vi "lookupImage.vi"(8 "error in (no error)":errorcluster, 11 "ImageStreamViewer in":refnum<class "ImageStreamViewer.lvclass">) -> (0 "error out":errorcluster, 3 "ImageStreamViewer out":refnum<class "ImageStreamViewer.lvclass">)   [LabVIEW 2009, in "Views.lvlib" / "Camera.lvlib" / "ImageStreamViewer.lvclass"]
uses:
  ImageStreamViewer.lvclass
  ImageStreamViewer.lvclass/ImageStreamViewer.ctl
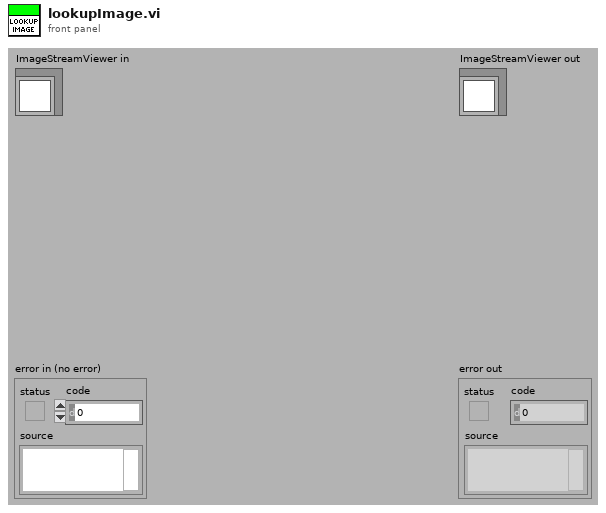
[diagram p1: front panel]
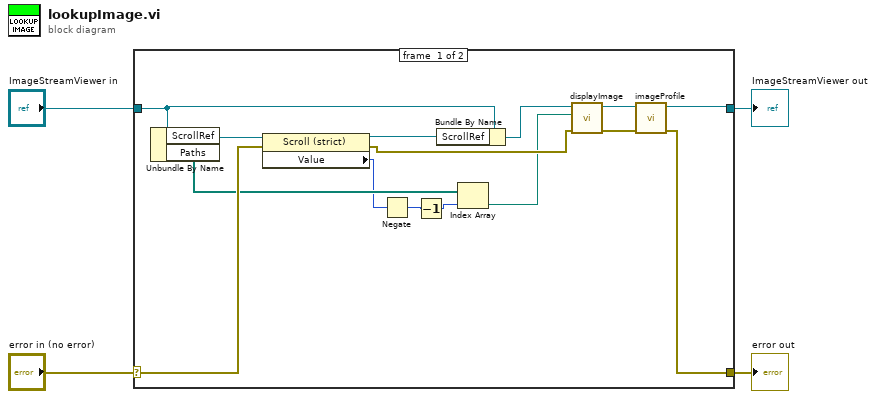
[diagram p0: block diagram]
diagram:
  n1 = case shown="No Error" "error in (no error)" {
    selector: "error in (no error)" -> [w18 w21]
    tunnel: [w5 w21] -> w3
    tunnel: [w6 w20] -> w1
    tunnel: "ImageStreamViewer in" -> [w12 w20]
    frame #0 {
      n2 = Unbundle By Name(w12) -> ("ScrollRef"=w19:refnum<vi>, "Paths"=w17:path[])
      n3 = property class="Scroll (strict)"(reference=w19, error in=w18) -> (reference out=w13:refnum<vi>, error out=w10:errorcluster, "Value"=w14:i32)
      n4 = Negate(x=w14) -> (-x=w16:i32)
      n5 = Decrement(x=w16) -> (x-1=w15:i32)
      n6 = Bundle By Name(cluster=w12, "ScrollRef"=w13) -> (w11:refnum<class "ImageStreamViewer.lvclass">)
      n7 = Index Array(array=w17, index=w15) -> (element=w9:path)
      n8 = call "displayImage.vi"("error in (no error)"=w10, "Path"=w9, "ImageStreamViewer in"=w11) -> ("error out"=w7:errorcluster, "ImageStreamViewer out"=w8:refnum<class "ImageStreamViewer.lvclass">)  [unwired: 7 in]
      n9 = call "imageProfile.vi"("error in (no error)"=w7, "ImageStreamViewer in"=w8) -> ("error out"=w5:errorcluster, "ImageStreamViewer out"=w6:refnum<class "ImageStreamViewer.lvclass">)  [unwired: 8 in]
    }
    frame #1 {
    }
  }
  "error out" <- w3
  "ImageStreamViewer out" <- w1
